vi "RPC Method package_service_method.vi"(3 "error in (no error)":errorcluster, 4 "gRPCid in":T1, 5 "ServiceClass in":refnum<class "ServiceImpl Template.lvclass">) -> (0 "error out":errorcluster, 1 "gRPCid out":T1, 2 "ServiceClass out":refnum<class "ServiceImpl Template.lvclass">)   [LabVIEW 2019, in "ServiceImpl Template.lvclass"]
uses:
  ServiceImpl Template.lvclass
  <vilib>/gRPC/LabVIEW gRPC Library/Shared/grpcId.ctl
  <vilib>/gRPC/LabVIEW gRPC Library/Server API/typeDefs/gRPC Status Code.ctl
  <vilib>/gRPC/LabVIEW gRPC Library/grpc-lvsupport-release.lvlib
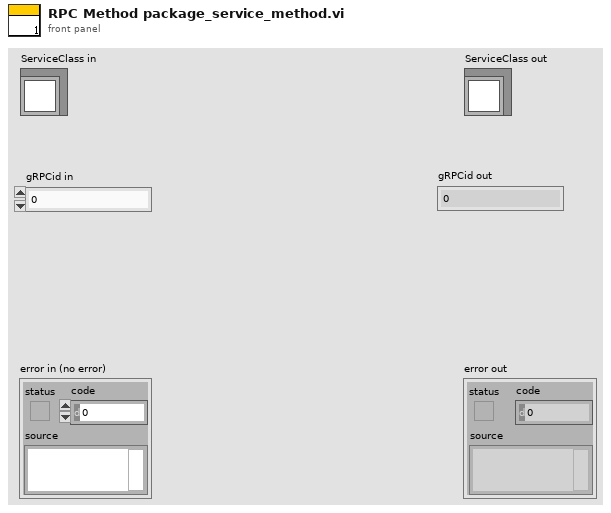
[diagram p1: front panel]
types:
  T1 = typedef "grpc-lvsupport-release.lvlib/grpcId.ctl" = u64
  T2 = typedef "grpc-lvsupport-release.lvlib/gRPC Status Code.ctl" = enum16{"OK", "CANCELLED", "UNKNOWN", "INVALID_ARGUMENT", "DEADLINE_EXCEEDED", "NOT_FOUND", "ALREADY_EXISTS", "PERMISSION_DENIED", "RESOURCE_EXHAUSTED", "FAILED_PRECONDITION", "ABORTED", "OUT_OF_RANGE", "UNIMPLEMENTED", "INTERNAL", "UNAVAILABLE", "DATA_LOSS", "UNAUTHENTICATED"}
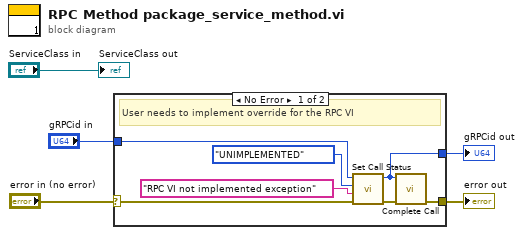
[diagram p0: block diagram]
diagram:
  n1 = case shown="No Error" "error in (no error)" {
    selector: "error in (no error)" -> [w10 w14]
    tunnel: [w6 w14] -> w4
    tunnel: [w7 w13] -> w2
    tunnel: "gRPCid in" -> [w12 w13]
    frame No Error {
      # "User needs to implement override for the RPC VI"
      n2 = call <vilib>:"Set Call Status.vi"("error in"=w10, "Details"="RPC VI not implemented exception", "Status Code"=gRPC_Status_Code."UNIMPLEMENTED", "gRPCid in"=w12) -> ("error out"=w8:errorcluster, "gRPCid out"=w7:T1)  [unwired: 6 in]
      n3 = call <vilib>:"Complete Call.vi"("gRPCid"=w7, "error in"=w8) -> ("error out"=w6:errorcluster)  [unwired: 8 in]
    }
    frame Error {
    }
  }
  "error out" <- w4
  "gRPCid out" <- w2
  "ServiceClass out" <- "ServiceClass in"
